vi "IDE_Example.vi"() -> ()   [LabVIEW 2020]
uses:
  Subs/ColorText/Code.xctl
  Subs/Console XCtrl/Console_Xctrl.xctl
  Subs/Server XCtrl/Server.xctl
panel:
  in  "Clean":bool
  in  "PC Save":bool
  in  "PC path":path
  in  "Files":bool
  in  "Server":bool
  in  "Help":bool
  in  "Server":path(xcontrol)=path "/Users/crogers/GitHub/Summer2020/LabVIEWCode/Servers/Jens.vi"
  out "REPL":string(xcontrol)
  in  "Clear":bool
  in  "Save":bool
  in  "Stop":bool
  in  "Run":bool
  in  "Name":string="code.py"
  in  "Code":string(xcontrol)="import os\n\nfor i in range(10):\n     print(i)\n"
  # "¨Processor"
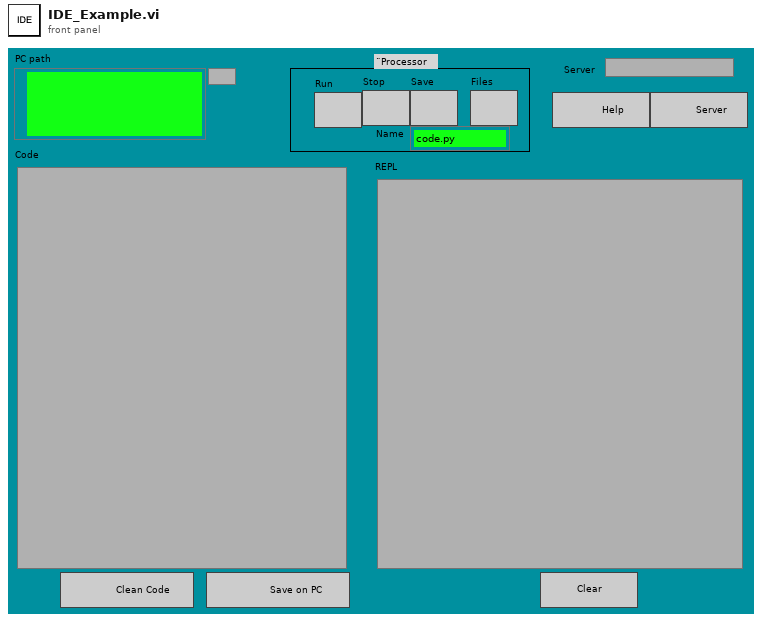
[diagram p1: front panel]
types:
  T1 = cluster{"Quote":u32, "Comment":u32, "Python":u32, "Text":u32, "Triple Quote":u32, "function":u32, "Line numbers":u32, "REPL Err":u32, "REPL Text":u32, "Text Bkgd":u32, "REPL Bkgd":u32}
  T2 = enum8{"Enabled", "Disabled", "Disabled and Grayed Out"}
  T3 = typedef "eventvkey.ctl" = enum16{"ASCII", "Enter", "Return", "Shift", "Ctrl", "Alt", "Cmd", "Opt", "Caps", "NumLock", "Clear", "Break", "Up", "Down", "Left", "Right", "Insert", "Delete", "Home", "End", "PageUp", "PageDown", "Escape", "Help", "Pause", "ScrollLock", "F1", "F2", "F3", "F4", "F5", "F6", "F7", "F8", "F9", "F10", "F11", "F12", "F13", "F14", "F15", "F16", "F17", "F18", "F19", "F20", "F21", "F22", "F23", "F24", "Play", "VolumeUp", "VolumeDown", "Mute", "Two Byte Char"}
  T4 = cluster{"Shift":bool, "Ctrl":bool, "Alt":bool, "Cmd":bool, "Opt":bool}
  T5 = cluster{"Char":i16, "VKey":T3, "PlatMods":cluster{"Shift":bool, "Ctrl":bool, "Alt":bool, "Cmd":bool, "Opt":bool}}
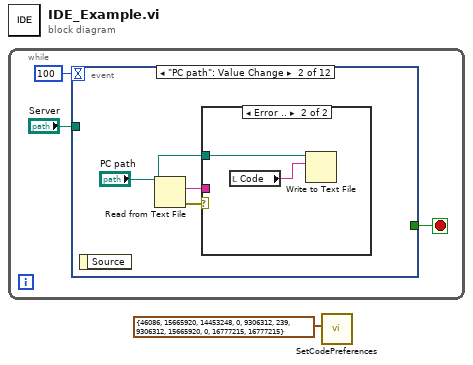
[diagram p0: block diagram]
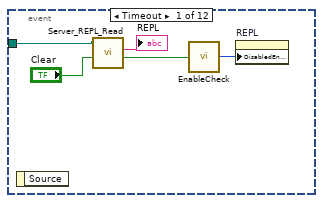
[diagram p2: hidden frame]
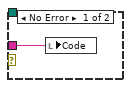
[diagram p3: hidden frame]
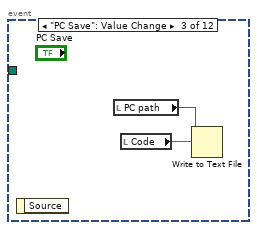
[diagram p4: hidden frame]
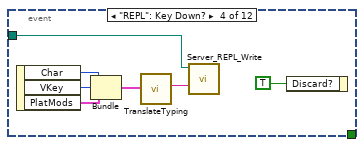
[diagram p5: hidden frame]
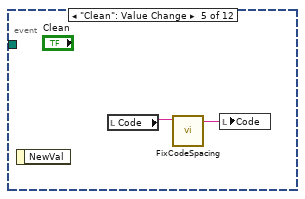
[diagram p6: hidden frame]
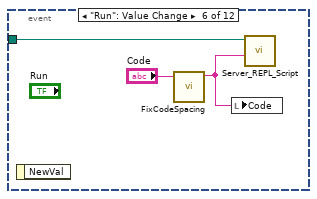
[diagram p7: hidden frame]
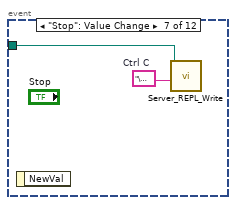
[diagram p8: hidden frame]
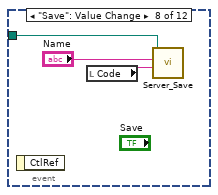
[diagram p9: hidden frame]
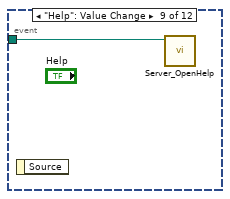
[diagram p10: hidden frame]
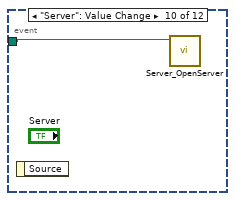
[diagram p11: hidden frame]
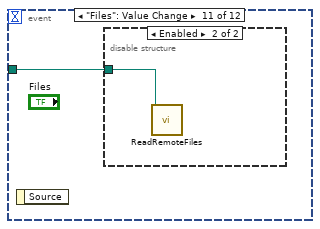
[diagram p12: hidden frame]
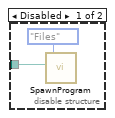
[diagram p13: hidden frame]
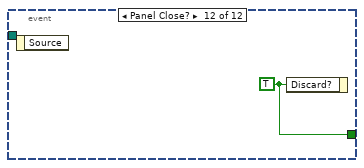
[diagram p14: hidden frame]
diagram:
  n1 = while {
    stop <- w3 stop-if-true
    n2 = event shown="[1] \"PC path\": Value Change" {
      selector: _ -> [_ _ _ _ _ _ _ _ _ _ _ _]
      dyn-events: _ -> [_ _ _ _ _ _ _ _ _ _ _ _]
      timeout: 100 -> [_ _ _ _ _ _ _ _ _ _ _ _]
      tunnel: [_ _ _ _ _ _ _ _ _ _ _ w41] -> w3
      tunnel: "Server" -> [w7 _ _ w18 _ w28 w30 w32 w35 w36 w37 _]
      event Timeout {
        n3 = event-data() -> ()  [unwired: 1 in, 1 out]
        n4 = call "Server_REPL_Read.vi"("Clear"="Clear", "Server"=w7) -> ("Running?"=w8:bool, "REPL"=→"REPL":string)  [unwired: 7 in, 1 out]
        n5 = call "EnableCheck.vi"("Enable?"=w8) -> ("Enum"=w9:T2)
        n6 = property on="REPL" class="Console_Xctrl (strict)"("DisabledEnum"=w9) -> ()  [unwired: 2 in, 2 out]
      }
      event "PC path": Value Change {
        n7 = event-data() -> ()  [unwired: 1 in, 1 out]
        n8 = Read from Text File(file (use dialog)="PC path") -> (text=w11:string, error out=w12:errorcluster)  [unwired: 3 in, 2 out]
        n9 = case shown="Error .." w12 {
          tunnel: w11 -> [w13 _]
          tunnel: "PC path" -> [_ w15]
          frame No Error {
            n10 = local write "Code"(w13) -> ()
          }
          frame Error {
            n11 = local read "Code"() -> (w14:string)
            n12 = Write to Text File(file (use dialog)=w15, text=w14) -> ()  [unwired: 2 in, 3 out]
          }
        }
      }
      event "PC Save": Value Change {
        n13 = event-data() -> ()  [unwired: 1 in, 1 out]
        n14 = local read "PC path"() -> (w17:path)
        n15 = local read "Code"() -> (w16:string)
        n16 = Write to Text File(file (use dialog)=w17, text=w16) -> ()  [unwired: 2 in, 3 out]
      }
      event "REPL": Key Down? {
        n17 = event-data() -> ("Char"=w23:i16, "VKey"=w22:T3, "PlatMods"=w20:T4)  [unwired: 1 in]
        n18 = Bundle("Char"=w23, "VKey"=w22, "PlatMods"=w20) -> (w24:T5)  [unwired: 1 in]
        n19 = call "TranslateTyping.vi"("Cluster"=w24) -> ("key"=w19:string)  [unwired: 10 in]
        n20 = call "Server_REPL_Write.vi"("Code"=w19, "Server"=w18) -> ()  [unwired: 9 in, 1 out]
        n21 = event-data("Discard?"=TRUE) -> ()  [unwired: 1 in, 1 out]
      }
      event "Clean": Value Change {
        n22 = event-data() -> ()  [unwired: 1 in, 1 out]
        n23 = local read "Code"() -> (w25:string)
        n24 = call "FixCodeSpacing.vi"("Code"=w25) -> ("Cleaned"=w26:string)  [unwired: 10 in]
        n25 = local write "Code"(w26) -> ()
      }
      event "Run": Value Change {
        n26 = event-data() -> ()  [unwired: 1 in, 1 out]
        n27 = call "FixCodeSpacing.vi"("Code"="Code") -> ("Cleaned"=w27:string)  [unwired: 10 in]
        n28 = local write "Code"(w27) -> ()
        n29 = call "Server_REPL_Script.vi"("Code"=w27, "Server"=w28) -> ()  [unwired: 9 in, 1 out]
      }
      event "Stop": Value Change {
        w31 = "\u0003"  # Ctrl C
        n30 = event-data() -> ()  [unwired: 1 in, 1 out]
        n31 = call "Server_REPL_Write.vi"("Code"=w31, "Server"=w30) -> ()  [unwired: 9 in, 1 out]
      }
      event "Save": Value Change {
        n32 = event-data() -> ()  [unwired: 1 in, 1 out]
        n33 = local read "Code"() -> (w34:string)
        n34 = call "Server_Save.vi"("Code"=w34, "Name"="Name", "Server"=w32) -> ()  [unwired: 8 in, 1 out]
      }
      event "Help": Value Change {
        n35 = event-data() -> ()  [unwired: 1 in, 1 out]
        n36 = call "Server_OpenHelp.vi"("Server"=w35) -> ()  [unwired: 10 in, 1 out]
      }
      event "Server": Value Change {
        n37 = event-data() -> ()  [unwired: 1 in, 1 out]
        n38 = call "Server_OpenServer.vi"("Server"=w36) -> ()  [unwired: 10 in, 1 out]
      }
      event "Files": Value Change {
        n39 = event-data() -> ()  [unwired: 1 in, 1 out]
        n40 = disable-structure shown="Enabled" {
          disable-tunnel: w37 -> [w38 w40]
          frame Disabled {
            n41 = call "SpawnProgram.vi"("Server"=w38, "Dialog"=enum16{"Help", "Files"}."Files") -> ()  [unwired: 10 in]
          }
          frame Enabled {
            n42 = call "ReadRemoteFiles.vi"("Server"=w40) -> ()  [unwired: 11 in]
          }
        }
      }
      event Panel Close? {
        w41 = TRUE ("Discard?")
        n43 = event-data() -> ()  [unwired: 1 in, 1 out]
        n44 = event-data("Discard?"=w41) -> ()  [unwired: 1 in, 1 out]
      }
    }
  }
  n45 = call "SetCodePreferences.vi"("Color choices"=T1 {"Quote"=46086, "Comment"=15665920, "Python"=14453248, "Text"=0, "Triple Quote"=9306312, "function"=239, "Line numbers"=9306312, "REPL Err"=15665920, "REPL Text"=0, "Text Bkgd"=16777215, "REPL Bkgd"=16777215}) -> ()  [unwired: 11 in]
